vi "XuLyStringData.vi"(4 "error IN":errorcluster, 5 "String":string) -> (0 "error out":errorcluster, 1 "Return State":T2, 2 "output cluster 2":T1)   [LabVIEW 2017]
uses:
  controls/STATE_MK4DUERETURNSTATE.ctl
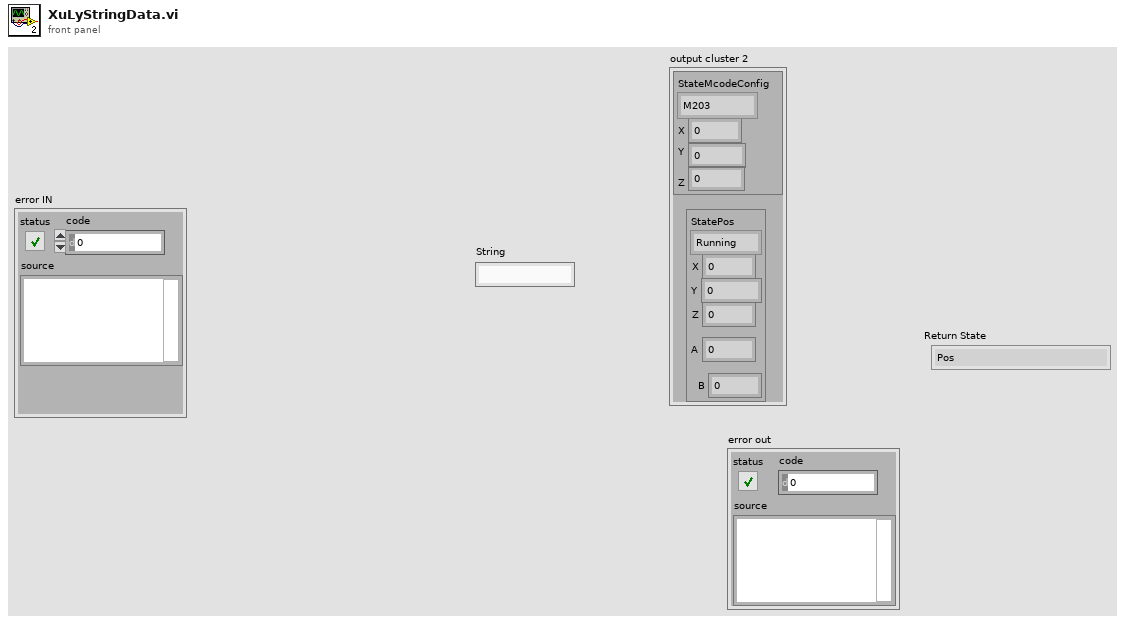
[diagram p1: front panel]
types:
  T1 = cluster{"OUTCONFIG":cluster{"StateMcodeConfig":enum16{"M203", "M201", "M92", "M3001"}, "X":dbl, "Y":dbl, "Z":dbl}, "outPOS":cluster{"StatePos":enum16{"Running", "Waiting", "Pos", "IDLE"}, "X":dbl, "Z":dbl, "Y":dbl, "A":dbl, "B":dbl}}
  T2 = typedef "STATE_MK4DUERETURNSTATE.ctl" = enum16{"Pos", "Config", "Echo", "OK", "Step", "Error"}
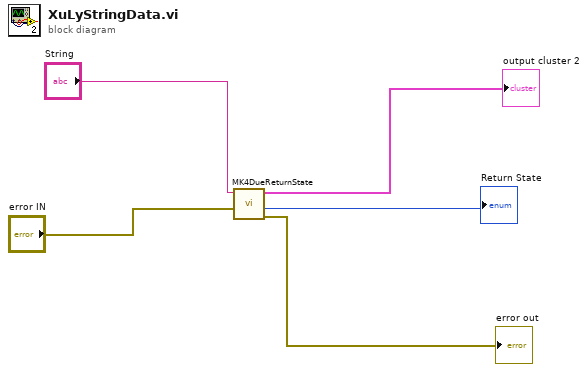
[diagram p0: block diagram]
diagram:
  n1 = call "MK4DueReturnState.vi"("error IN"="error IN", "String IN"="String") -> ("error out"=→"error out":errorcluster, "Return State 2"=→"Return State":T2, "output cluster"=→"output cluster 2":T1)  [unwired: 4 in]
